vi "Convert mouse to teleop command.vi"(8 "error in (no error)":errorcluster, 9 "key mode":enum16{"RELATIVE", "ABSOLUTE"}(ring)=enum."ABSOLUTE", 10 "Teleop command in":T1, 11 "Mouse in":refnum<k1>) -> (0 "error out":errorcluster, 2 "Teleop command out":T1, 3 "Mouse out":refnum<k1>)   [LabVIEW 2012]
uses:
  Teleop command.ctl
  <vilib>/Utility/inputDevices.llb/mouseAcquire.vi
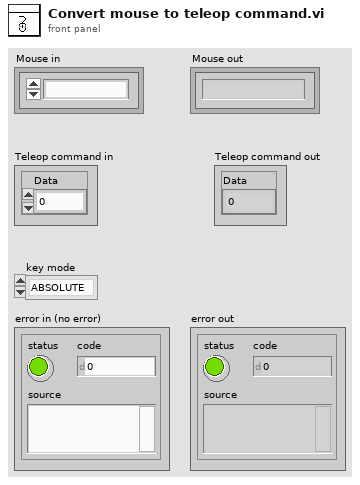
[diagram p1: front panel]
types:
  T1 = typedef "Teleop command.ctl" = cluster{"Data":dbl}
  T2 = cluster{"Horizontal":i32, "Vertical":i32, "Scrolling":i32}
  T3 = cluster{"button 1":bool, "button 2":bool, "button 3":bool, "button 4":bool}
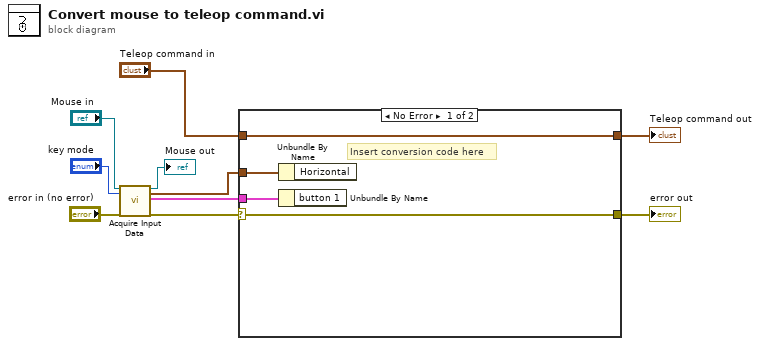
[diagram p0: block diagram]
diagram:
  n1 = call-poly <vilib>:"Acquire Input Data.vi"("device ID"="Mouse in", "key mode"="key mode", "error in (no error)"="error in (no error)") -> ("device ID"=→"Mouse out":refnum<k1>, "axis info"=w3:T2, "button info"=w2:T3, "error out"=w7:errorcluster)  [unwired: 13 in]
  n2 = case shown="No Error" w7 {
    selector: w7 -> [w14 w16]
    tunnel: [w14 w16] -> w6
    tunnel: "Teleop command in" -> [w11 w15]
    tunnel: [w11 w15] -> w4
    tunnel: w3 -> [w13 _]
    tunnel: w2 -> [w12 _]
    frame No Error {
      # "Insert conversion code here"
      n3 = Unbundle By Name(w13) -> ()  [unwired: 1 out]
      n4 = Unbundle By Name(w12) -> ()  [unwired: 1 out]
    }
    frame Error {
    }
  }
  "Teleop command out" <- w4
  "error out" <- w6
